vi "VI Tree.vi"   [LabVIEW 2019, in "Lake Shore 325.lvlib"]
doc: "This is the instrument driver for the Lake Shore Model 325 Temperature Controller. The VI Tree displays all the user-callable VIs of the instrument driver in an organized table."
uses:
  Lake Shore 325.lvlib
  Data/Sensor Data (Single Reading).vi
panel:
  # "© 2006 Lake Shore Cryotronics Inc.  ALL RIGHTS RESERVED."
  # "SEE DIAGRAM\nFOR VI TREE."
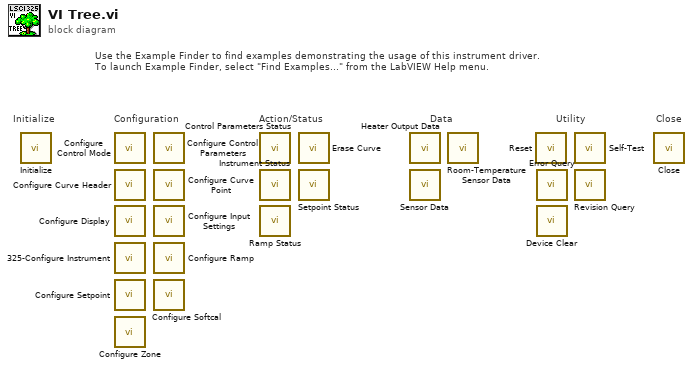
[diagram p0: block diagram]
diagram:
  # "Use the Example Finder to find examples demonstrating the usage of this instrument driver.\nTo launch Example Finder, select \"Find Examples...\" from the LabVIEW Help menu."
  # "Configuration"
  # "Utility"
  # "Data"
  # "Action/Status"
  # "Close"
  # "Initialize"
  n1 = call "Initialize.vi"() -> ()  [unwired: 10 in, 2 out]
  n2 = call "Configure Control Mode.vi"() -> ()  [unwired: 14 in, 2 out]
  n3 = call "Configure Curve Header.vi"() -> ()  [unwired: 14 in, 2 out]
  n4 = call "Configure Display.vi"() -> ()  [unwired: 14 in, 2 out]
  n5 = call "325-Configure Instrument.vi"() -> ()  [unwired: 14 in, 2 out]
  n6 = call "Configure Setpoint.vi"() -> ()  [unwired: 14 in, 2 out]
  n7 = call "Configure Zone.vi"() -> ()  [unwired: 13 in, 3 out]
  n8 = call "Configure Control Parameters.vi"() -> ()  [unwired: 14 in, 2 out]
  n9 = call "Configure Curve Point.vi"() -> ()  [unwired: 14 in, 2 out]
  n10 = call "Configure Input Settings.vi"() -> ()  [unwired: 14 in, 2 out]
  n11 = call "Configure Ramp.vi"() -> ()  [unwired: 14 in, 2 out]
  n12 = call "Configure Softcal.vi"() -> ()  [unwired: 14 in, 2 out]
  n13 = call "Control Parameters Status.vi"() -> ()  [unwired: 7 in, 9 out]
  n14 = call "Instrument Status.vi"() -> ()  [unwired: 6 in, 6 out]
  n15 = call "Ramp Status.vi"() -> ()  [unwired: 7 in, 5 out]
  n16 = call "Erase Curve.vi"() -> ()  [unwired: 10 in, 2 out]
  n17 = call "Setpoint Status.vi"() -> ()  [unwired: 9 in, 3 out]
  n18 = call "Heater Output Data.vi"() -> ()  [unwired: 9 in, 3 out]
  n19 = call-poly "Sensor Data.vi"() -> ()  [unwired: 9 in, 3 out]
  n20 = call "Room-Temperature Sensor Data.vi"() -> ()  [unwired: 9 in, 3 out]
  n21 = call "Reset.vi"() -> ()  [unwired: 10 in, 2 out]
  n22 = call "Error Query.vi"() -> ()  [unwired: 9 in, 3 out]
  n23 = call "Device Clear.vi"() -> ()  [unwired: 10 in, 2 out]
  n24 = call "Self-Test.vi"() -> ()  [unwired: 8 in, 4 out]
  n25 = call "Revision Query.vi"() -> ()  [unwired: 6 in, 6 out]
  n26 = call "Close.vi"() -> ()  [unwired: 11 in, 1 out]
